vi "Read Interlock Values.vi"(8 "error in (no error)":errorcluster, 11 "Door Interlocks in":refnum<class "Door Interlocks.lvclass">) -> (0 "error out":errorcluster, 2 "Interlock Values":T1)   [LabVIEW 2020, in "Door Interlocks.lvclass"]
uses:
  Door Interlocks.lvclass
  Interlock Values.ctl
  Mode of Operation.ctl
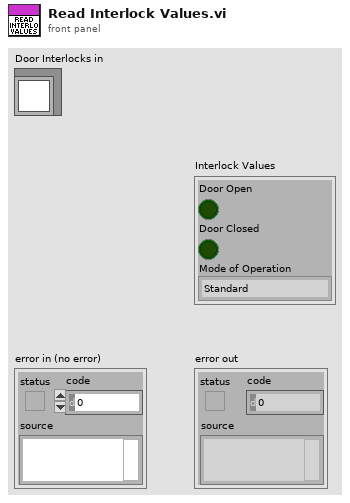
[diagram p1: front panel]
types:
  T1 = typedef "Door Interlocks.lvclass/Interlock Values.ctl" = cluster{"Door Open":bool, "Door Closed":bool, "Mode of Operation":T2}
  T2 = typedef "Door Interlocks.lvclass/Mode of Operation.ctl" = enum16{"Standard", "Interlock Override"}
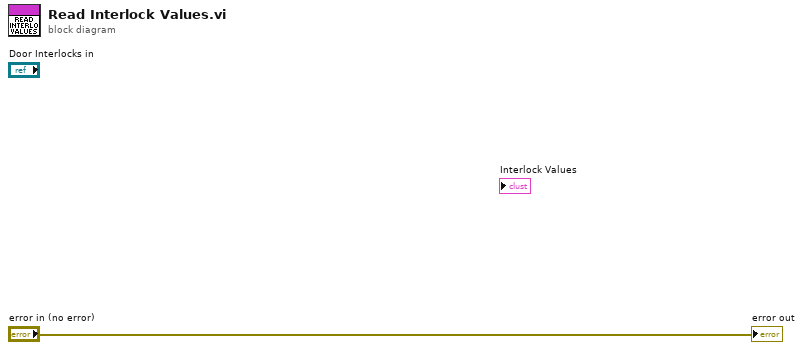
[diagram p0: block diagram]
diagram:
  "error out" <- "error in (no error)"
